vi "Format NN Parameter.vi"(1 "nn1":dbl) -> (0 "String":string)   [LabVIEW 2015]
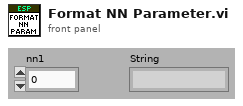
[diagram p1: front panel]
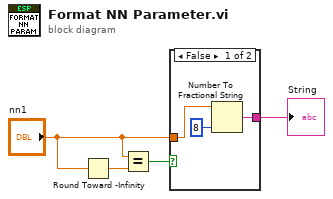
[diagram p0: block diagram]
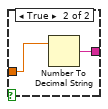
[diagram p2: hidden frame]
diagram:
  n1 = Round Toward -Infinity(1:"nn1") -> (0:w3:dbl)
  n2 = Equal?(x="nn1", y=w3) -> (x = y?=w1:bool)
  n3 = case shown="False" w1 {
    tunnel: [w6 w9] -> w4
    tunnel: "nn1" -> [w7 w8]
    frame False {
      n4 = Number To Fractional String(number=w7, precision (6)=i16 8) -> (F-format string=w6:string)  [unwired: 2 in]
    }
    frame True {
      n5 = Number To Decimal String(number=w8) -> (decimal integer string=w9:string)  [unwired: 1 in]
    }
  }
  "String" <- w4
